vi "1L25_conv_unite_temp.vi"(1 "Valeur":dbl, 2 "Unité de départ":u16, 3 "Unité pour conversion":u16, 4 "Refnum":refnum<vi>) -> (0 "Valeur fin":dbl)   [LabVIEW 2010, in "lv_01.lvlib"]
doc: "L'utilisateur sélectionne l'unité de la température saisie dans la commande Valeur. Le programme fait la conversion de la valeur selon l'unité pour conversion sélectionnée.\nPour utiliser ce sous-VI, activer le sous-titre pour l'indicateur de la température en sortie, puis avec un clic droit sur la commande, créer une référence que vous allez câbler sur l'entrée Refnum"
uses:
  lv_01.lvlib
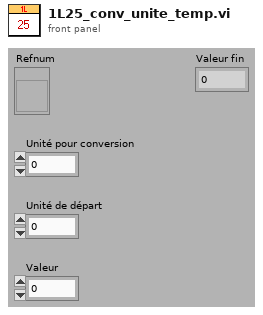
[diagram p1: front panel]
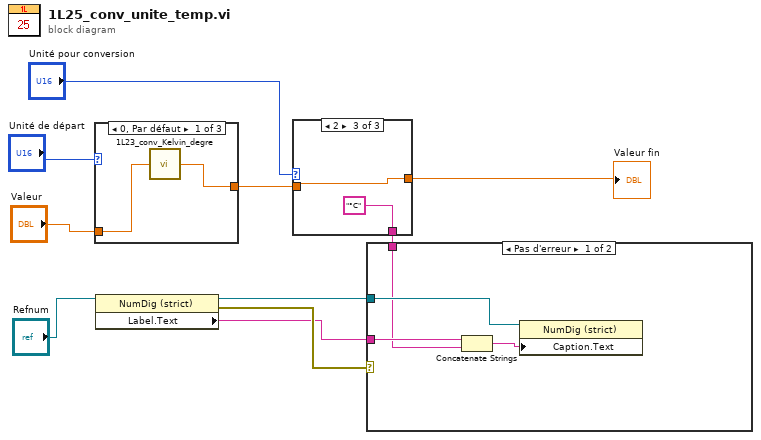
[diagram p0: block diagram]
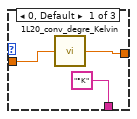
[diagram p3: hidden frame]
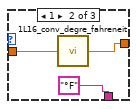
[diagram p4: hidden frame]
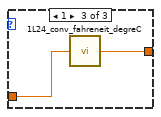
[diagram p6: hidden frame]
diagram:
  n1 = case shown="0, Par défaut" "Unité de départ" {
    tunnel: "Valeur" -> [w12 w13 w15]
    tunnel: [w11 w13 w14] -> w10
    frame 0, Default {
      n2 = call "1L23_conv_Kelvin_degre.vi"("Deg K"=w12) -> ("Deg C"=w11:dbl)
    }
    frame 2 {
    }
    frame 1 {
      n3 = call "1L24_conv_fahreneit_degreC.vi"("Deg F"=w15) -> ("Deg C"=w14:dbl)
    }
  }
  n4 = property on="Nœud de propriété" class="NumDig (strict)"(reference="Refnum") -> (reference out=w3:refnum<vi>, error out=w6:errorcluster, "Label.Text"=w4:string)  [unwired: 1 in]
  n5 = case shown="2" "Unité pour conversion" {
    tunnel: w10 -> [w17 w21 w23]
    tunnel: [w16 w20 w23] -> w2
    tunnel: ["°K" ("Étiquette.Texte") "°F" ("Étiquette.Texte") "°C" ("Étiquette.Texte")] -> w1
    frame 0, Default {
      n6 = call "1L20_conv_degre_Kelvin.vi"("Deg C"=w17) -> ("Deg K"=w16:dbl)
    }
    frame 1 {
      n7 = call "1L16_conv_degre_fahreneit.vi"("Deg C"=w21) -> ("Deg F"=w20:dbl)
    }
    frame 2 {
    }
  }
  "Valeur fin" <- w2
  n8 = case shown="Pas d'erreur" w6 {
    tunnel: w4 -> [w26 _]
    tunnel: w3 -> [w25 _]
    tunnel: w1 -> [w24 _]
    frame No Error {
      n9 = Concatenate Strings(w26, w24) -> (w27:string)
      n10 = property on="Nœud de propriété" class="NumDig (strict)"(reference=w25, "Caption.Text"=w27) -> ()  [unwired: 1 in, 2 out]
    }
    frame Error {
    }
  }
